vi "3.8-TCP Receive Server.vi"() -> ()   [LabVIEW 2010]
doc: "Sends a specified waveform through a TCP port. The VI first listens for a connection and, once established, sends the number of bytes to be sent followed by the data. After the data is sent, the VI waits for an 'all received' signal from the client and then breaks the connection.\n\n<B>Note:</B> Requires the Data Client.vi located in the same library as this VI."
uses:
  4-High Neurons/4.0-Timing Badass.ctl
  3.0 Flow Control/3.0 List of Loops.ctl
  3.0-Global.vi
  3.0 - Functional Array Holding Global.vi
panel:
  out "Variant Cast":T1
  out "GUI":T1
  in  "Port":u16=53483 min=1025 step=1
  # "Instructions:\n1. Open the Data Client.vi\n2. Run This VI first.\n3. Run the Data Client.vi Second.\n4. Adjust the # of Points Function, and Noise Level controls.\n5. Observe the Chart on the Data Client.vi.\n6. Stop This VI. The Data Client.vi will time out and stop."
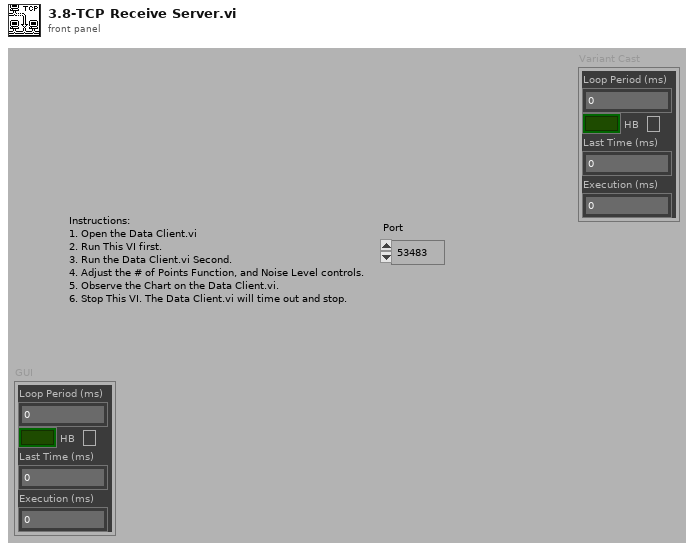
[diagram p1: front panel]
types:
  T1 = typedef "4.0-Timing Badass.ctl" = cluster{"Loop Period (ms)":u32, "HB":bool, "Last Time (ms)":u32, "Execution (ms)":u32}
  T2 = typedef "3.0 List of Loops.ctl" = enum16{"3.0 State Update", "3.0 GUI", "3.1 Act", "3.1 4.7.1 Act UDP", "3.1 Joystick", "3.2 Where", "3.2 4.7.2 Where UDP", "3.3 What", "3.3 4.7.3 What UDP", "3.4 How", "3.4 4.7.4 How UDP", "3.5 Limbic", "3.8 TCP", "3.6 Cerebellum", "3.8 TCP Act"}
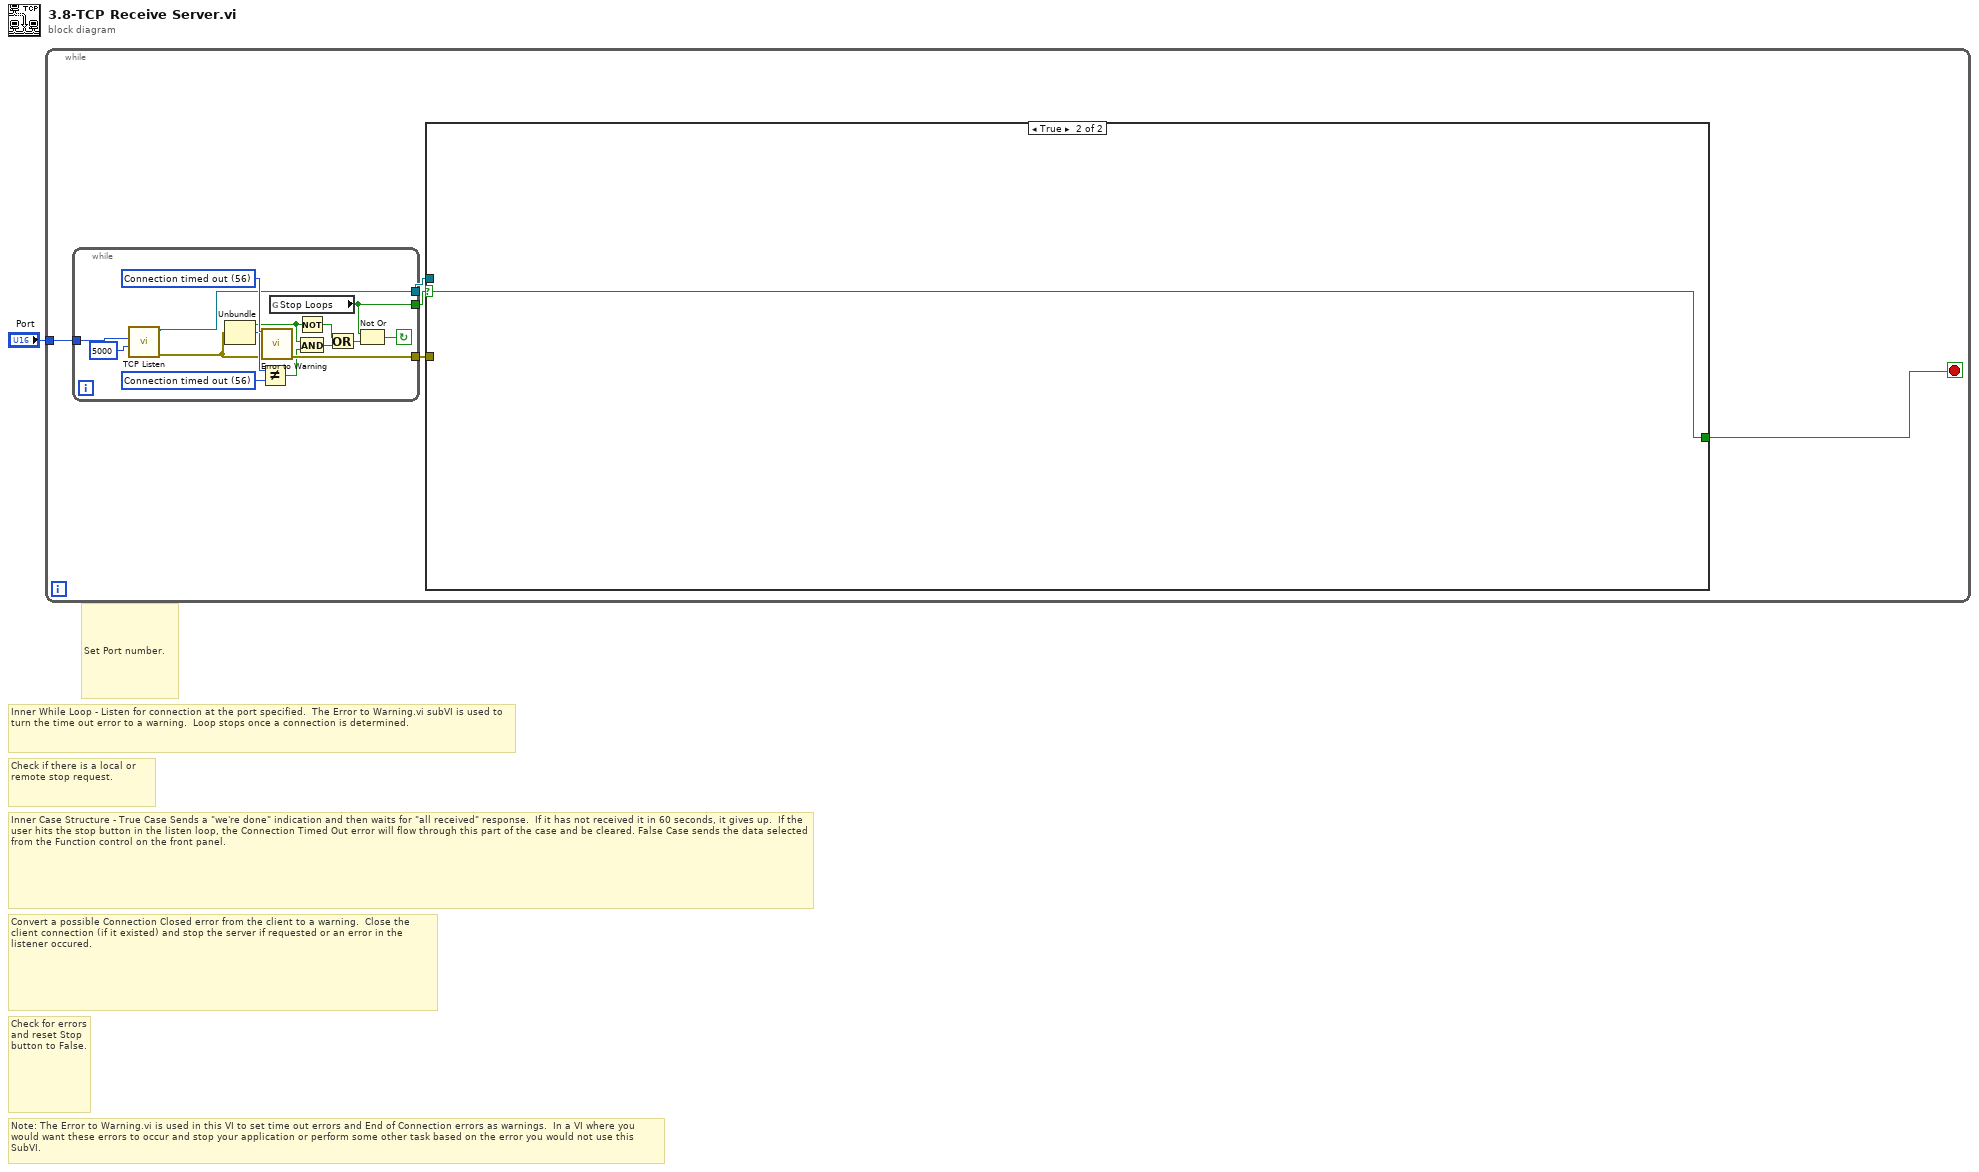
[diagram p0: block diagram]
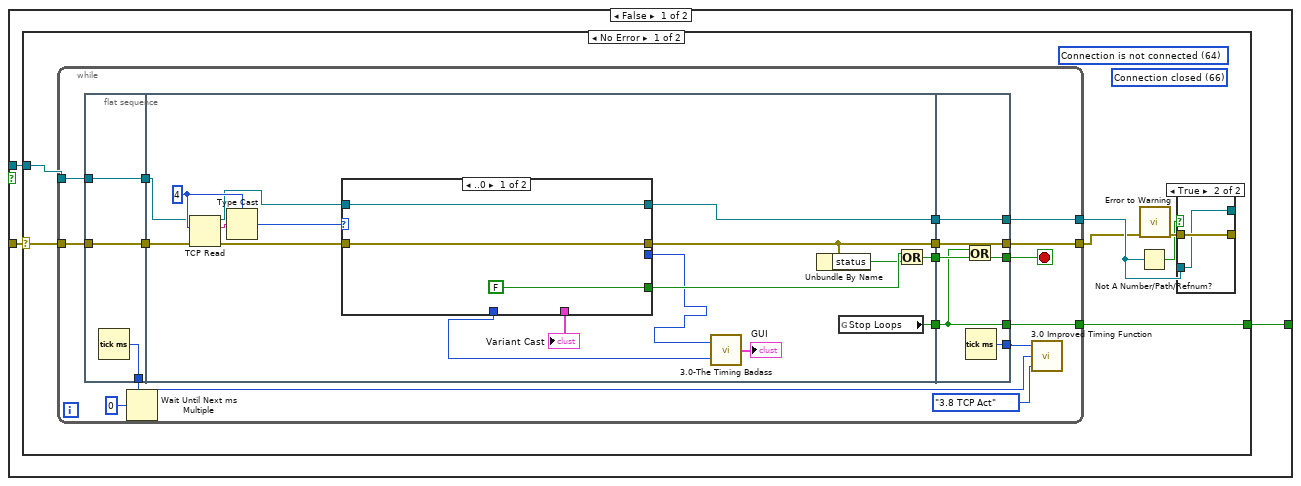
[diagram p2: hidden frame]
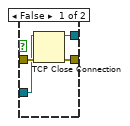
[diagram p3: hidden frame]
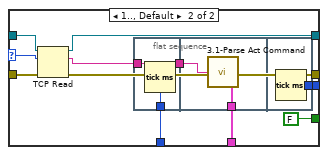
[diagram p4: hidden frame]
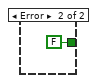
[diagram p5: hidden frame]
diagram:
  # "Check for errors\nand reset Stop \nbutton to False."
  # "Inner Case Structure - True Case Sends a \"we're done\" indication and then waits for \"all received\" response.  If it has not received it in 60 seconds, it gives up.  If the user hits the stop button in the listen loop, the Connection Timed Out error will flow through this part of the case and be cleared. False Case sends the data selected from the Function control on the front panel."
  # "Check if there is a local or remote stop request."
  # "Set Port number."
  # "Inner While Loop - Listen for connection at the port specified.  The Error to Warning.vi subVI is used to turn the time out error to a warning.  Loop stops once a connection is determined."
  # "Note: The Error to Warning.vi is used in this VI to set time out errors and End of Connection errors as warnings.  In a VI where you would want these errors to occur and stop your application or perform some other task based on the error you would not use this SubVI."
  # "Convert a possible Connection Closed error from the client to a warning.  Close the client connection (if it existed) and stop the server if requested or an error in the listener occured."
  n1 = while {
    tunnel: "Port" -> [w6]
    stop <- w2 stop-if-true
    n2 = while {
      tunnel: [w9] -> w3
      tunnel: [w18] -> w4
      tunnel: [w8] -> w5
      tunnel: w6 -> [w21]
      stop <- w19 continue-if-true
      w16 = 56 items=["No Error", "Argument Error", "Memory Full", "Out of Zone", "End of File", "File Already Open", "Generic File IO Error", "File Not Found", "File Permission Error", "Disk Full", "Duplicate Path", "Too Many Files Open", "Not Enabled", "Resource File Not Found", "Cannot Add Resource", "Resource Not Found", "Image Not Found", "Image Memory Error", "Pen Does Not Exist", "Config Bad Type", "Config Token Not Found", "Config Parse Error", "Config Memory Error", "Bad External Code Format", "Bad External Code Offset", "External Code Not Present", "Null Window", "Destroy Window Mixup", "Null Menu", "Print Aborted", "Bad Print Record", "Print Driver Error", "Windows Error During Print", "Memory Error During Print", "Print Dialog Error", "Generic Print Error", "Invalid Device Refnum", "Device Not Found", "Device Parameter Error", "Device Unit Error", "Can't Open Device", "Device Call Aborted", "Generic Error", "Cancelled By User", "Object ID Too Low", "Object ID Too High", "Object Not In Heap", "Unknown Heap", "Bad DefProc ID", "DefProc Not In Table", "Message Out Of Range", "Null Method", "Unknown Message", "Manager Call Not Supported", "Bad address", "Connection In progress", "Connection timed out", "Connection is already in progress", "Network attribute not supported", "Network error", "Address in use", "System out of memory", "Connection aborted", "Connection refused", "Connection is not connected", "Connection is already connected", "Connection closed", "Initialize error (interapplication manager)", "Bad occurrence", "Wait on unbound occurrence handler", "Occurrence queue overflow", "Bad path", "Semaphore not signaled", "Unrecognized type (interapplication manager)"] ("1st Error to Convert")
      w17 = 56 items=["No Error", "Argument Error", "Memory Full", "Out of Zone", "End of File", "File Already Open", "Generic File IO Error", "File Not Found", "File Permission Error", "Disk Full", "Duplicate Path", "Too Many Files Open", "Not Enabled", "Resource File Not Found", "Cannot Add Resource", "Resource Not Found", "Image Not Found", "Image Memory Error", "Pen Does Not Exist", "Config Bad Type", "Config Token Not Found", "Config Parse Error", "Config Memory Error", "Bad External Code Format", "Bad External Code Offset", "External Code Not Present", "Null Window", "Destroy Window Mixup", "Null Menu", "Print Aborted", "Bad Print Record", "Print Driver Error", "Windows Error During Print", "Memory Error During Print", "Print Dialog Error", "Generic Print Error", "Invalid Device Refnum", "Device Not Found", "Device Parameter Error", "Device Unit Error", "Can't Open Device", "Device Call Aborted", "Generic Error", "Cancelled By User", "Object ID Too Low", "Object ID Too High", "Object Not In Heap", "Unknown Heap", "Bad DefProc ID", "DefProc Not In Table", "Message Out Of Range", "Null Method", "Unknown Message", "Manager Call Not Supported", "Bad address", "Connection In progress", "Connection timed out", "Connection is already in progress", "Network attribute not supported", "Network error", "Address in use", "System out of memory", "Connection aborted", "Connection refused", "Connection is not connected", "Connection is already connected", "Connection closed", "Initialize error (interapplication manager)", "Bad occurrence", "Wait on unbound occurrence handler", "Occurrence queue overflow", "Bad path", "Semaphore not signaled", "Unrecognized type (interapplication manager)"] ("1st Error to Convert")
      n3 = call <vilib>:"TCP Listen.vi"("timeout ms (wait forever: -1)"=5000, "port"=w21) -> ("error out"=w7:errorcluster, "connection ID"=w8:refnum<k5>)  [unwired: 6 in, 2 out]
      n4 = Unbundle(w7) -> ("status"=w14:bool, "code"=w15:i32)  [unwired: 1 out]
      n5 = Not Equal?(x=w15, y=w16) -> (x != y?=w13:bool)
      n6 = call <vilib>:"Error to Warning.vi"("1st Error to Convert"=w17, "error in"=w7) -> ("warning out"=w18:errorcluster)  [unwired: 13 in]
      n7 = global read "3.0-Global.vi" "Stop Loops"() -> (w9:bool)
      n8 = Not(x=w14) -> (.not. x?=w12:bool)
      n9 = And(x=w14, y=w13) -> (x .and. y?=w11:bool)
      n10 = Or(x=w12, y=w11) -> (x .or. y?=w10:bool)
      n11 = Not Or(1:w10, 2:w9) -> (0:w19:bool)
    }
    n12 = case shown="True" w3 {
      selector: w3 -> [_ w100]
      tunnel: w5 -> [w24 _]
      tunnel: w4 -> [w22 _]
      tunnel: [w23 w100] -> w2
      frame False {
        n13 = case shown="No Error" w22 {
          selector: w22 -> [w30 _]
          tunnel: w24 -> [w31 _]
          tunnel: [w29 FALSE] -> w23
          frame No Error {
            (unwired) 66 items=["No Error", "Argument Error", "Memory Full", "Out of Zone", "End of File", "File Already Open", "Generic File IO Error", "File Not Found", "File Permission Error", "Disk Full", "Duplicate Path", "Too Many Files Open", "Not Enabled", "Resource File Not Found", "Cannot Add Resource", "Resource Not Found", "Image Not Found", "Image Memory Error", "Pen Does Not Exist", "Config Bad Type", "Config Token Not Found", "Config Parse Error", "Config Memory Error", "Bad External Code Format", "Bad External Code Offset", "External Code Not Present", "Null Window", "Destroy Window Mixup", "Null Menu", "Print Aborted", "Bad Print Record", "Print Driver Error", "Windows Error During Print", "Memory Error During Print", "Print Dialog Error", "Generic Print Error", "Invalid Device Refnum", "Device Not Found", "Device Parameter Error", "Device Unit Error", "Can't Open Device", "Device Call Aborted", "Generic Error", "Cancelled By User", "Object ID Too Low", "Object ID Too High", "Object Not In Heap", "Unknown Heap", "Bad DefProc ID", "DefProc Not In Table", "Message Out Of Range", "Null Method", "Unknown Message", "Manager Call Not Supported", "Bad address", "Connection In progress", "Connection timed out", "Connection is already in progress", "Network attribute not supported", "Network error", "Address in use", "System out of memory", "Connection aborted", "Connection refused", "Connection is not connected", "Connection is already connected", "Connection closed", "Initialize error (interapplication manager)", "Bad occurrence", "Wait on unbound occurrence handler", "Occurrence queue overflow", "Bad path", "Semaphore not signaled", "Unrecognized type (interapplication manager)"] ("2nd Error to Convert")
            (unwired) 64 items=["No Error", "Argument Error", "Memory Full", "Out of Zone", "End of File", "File Already Open", "Generic File IO Error", "File Not Found", "File Permission Error", "Disk Full", "Duplicate Path", "Too Many Files Open", "Not Enabled", "Resource File Not Found", "Cannot Add Resource", "Resource Not Found", "Image Not Found", "Image Memory Error", "Pen Does Not Exist", "Config Bad Type", "Config Token Not Found", "Config Parse Error", "Config Memory Error", "Bad External Code Format", "Bad External Code Offset", "External Code Not Present", "Null Window", "Destroy Window Mixup", "Null Menu", "Print Aborted", "Bad Print Record", "Print Driver Error", "Windows Error During Print", "Memory Error During Print", "Print Dialog Error", "Generic Print Error", "Invalid Device Refnum", "Device Not Found", "Device Parameter Error", "Device Unit Error", "Can't Open Device", "Device Call Aborted", "Generic Error", "Cancelled By User", "Object ID Too Low", "Object ID Too High", "Object Not In Heap", "Unknown Heap", "Bad DefProc ID", "DefProc Not In Table", "Message Out Of Range", "Null Method", "Unknown Message", "Manager Call Not Supported", "Bad address", "Connection In progress", "Connection timed out", "Connection is already in progress", "Network attribute not supported", "Network error", "Address in use", "System out of memory", "Connection aborted", "Connection refused", "Connection is not connected", "Connection is already connected", "Connection closed", "Initialize error (interapplication manager)", "Bad occurrence", "Wait on unbound occurrence handler", "Occurrence queue overflow", "Bad path", "Semaphore not signaled", "Unrecognized type (interapplication manager)"] ("1st Error to Convert")
            n14 = while {
              tunnel: [w52] -> w26
              tunnel: [w51] -> w25
              tunnel: w31 -> [w50]
              tunnel: w30 -> [w49]
              tunnel: [w48] -> w29
              stop <- w53 stop-if-true
              n15 = flat-sequence {
                tunnel: w49 -> [w55]
                tunnel: w50 -> [w56]
                tunnel: [w56] -> w43
                tunnel: [w55] -> w42
                tunnel: [w54] -> w40
                tunnel: [w72] -> w47
                tunnel: [w58] -> w46
                tunnel: [w57] -> w45
                tunnel: [w63] -> w44
                tunnel: w43 -> [w65]
                tunnel: w42 -> [w64]
                tunnel: [w93] -> w48
                tunnel: [w96] -> w51
                tunnel: [w97] -> w52
                tunnel: [w94] -> w53
                tunnel: w47 -> [w98]
                tunnel: w46 -> [w97]
                tunnel: w45 -> [w96]
                tunnel: w44 -> [w93]
                tunnel: [w95] -> w41
                frame #0 {
                  n16 = Tick Count (ms)() -> (millisecond timer value=w54:u32)
                }
                frame #1 {
                  w71 = 4
                  n17 = TCP Read(connection ID=w65, bytes to read=w71, error in (no error)=w64) -> (connection ID out=w67:refnum<k5>, data out=w73:string, error out=w68:errorcluster)  [unwired: 2 out]
                  n18 = Type Cast(type=w71, x=w73) -> (*(type *) &x=w70:i32)
                  n19 = case shown="..0" w70 {
                    selector: w70 -> [_ w84]
                    tunnel: w68 -> [w74 w87]
                    tunnel: w67 -> [w76 w86]
                    tunnel: [w76 w85] -> w58
                    tunnel: [FALSE FALSE] -> w69
                    tunnel: [w74 w82] -> w57
                    tunnel: [_ w79] -> w61
                    tunnel: [_ w78] -> w60
                    tunnel: [_ w77] -> w59
                    frame ..0 {
                    }
                    frame 1.., Default {
                      n20 = TCP Read(connection ID=w86, bytes to read=w84, error in (no error)=w87) -> (connection ID out=w85:refnum<k5>, data out=w81:string, error out=w82:errorcluster)  [unwired: 2 out]
                      n21 = flat-sequence {
                        tunnel: w81 -> [w89]
                        tunnel: [w89] -> w80
                        tunnel: [w88] -> w78
                        tunnel: w80 -> [w91]
                        tunnel: [w90] -> w77
                        tunnel: [w92] -> w79
                        frame #0 {
                          n22 = Tick Count (ms)() -> (millisecond timer value=w88:u32)
                        }
                        frame #1 {
                          n23 = call "3.1-Parse Act Command.vi"("data out"=w91) -> ("GUI"=w90:T1)
                        }
                        frame #2 {
                          n24 = Tick Count (ms)() -> (millisecond timer value=w92:u32)
                        }
                      }
                    }
                  }
                  "Variant Cast" <- w59
                  n25 = call "3.0-The Timing Badass.vi"("Start"=w60, "End"=w61) -> ("Super Heart Beat"=→"GUI":T1)
                  n26 = Unbundle By Name(w57) -> ("status"=w66:bool)
                  n27 = global read "3.0-Global.vi" "Stop Loops"() -> (w63:bool)
                  n28 = Or(x=w69, y=w66) -> (x .or. y?=w72:bool)
                }
                frame #2 {
                  n29 = Or(x=w93, y=w98) -> (x .or. y?=w94:bool)
                  n30 = Tick Count (ms)() -> (millisecond timer value=w95:u32)
                }
              }
              n31 = Wait Until Next ms Multiple(millisecond multiple=u32 0) -> ()  [unwired: 1 out]
              n32 = call "3.0 Improved Timing Function.vi"("Loop"=3.0_List_of_Loops."3.8 TCP Act", "Start"=w40, "End"=w41) -> ()  [unwired: 1 in]
            }
            n33 = Not A Number/Path/Refnum?(number/path/refnum=w26) -> (NaN/Path/Refnum?=w27:bool)
            n34 = call <vilib>:"Error to Warning.vi"("error in"=w25) -> ("warning out"=w28:errorcluster)  [unwired: 14 in]
            n35 = case shown="True" w27 {
              tunnel: w28 -> [w35 w37]
              tunnel: w26 -> [w34 w36]
              tunnel: [w33 w37] -> _
              tunnel: [w32 w36] -> _
              frame False {
                n36 = TCP Close Connection(connection ID=w34, error in (no error)=w35) -> (connection ID out=w32:refnum<k5>, error out=w33:errorcluster)  [unwired: 1 in]
              }
              frame True {
              }
            }
          }
          frame Error {
          }
        }
      }
      frame True {
      }
    }
  }
